vi "Sequence Status.vi"(5 "Exists Locally":bool, 7 "Local Error":bool, 10 "Local CRC":u32, 11 "Sequence Status JSON":T2) -> (3 "Sequence Status":T1=enum."Unloaded")   [LabVIEW 2023, in "VolatusSeqGUI.lvlib" / "Sequencing Control.lvclass"]
uses:
  Sequencing Control.lvclass
  VolatusSeq/Sequence Status JSON.ctl
  Sequence Status.ctl
  Sequencing Control.lvclass/Sequencing Control.ctl
  VolatusSeq/VolatusSeq.lvlib
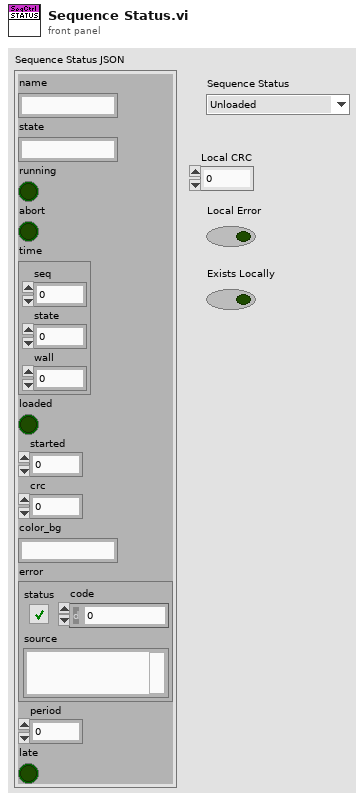
[diagram p1: front panel]
types:
  T1 = typedef "VolatusSeqGUI.lvlib/Sequencing Control.lvclass/Sequence Status.ctl" = enum16{"Unloaded Not Local", "Unloaded", "Load Error", "Loaded Good CRC", "Loaded Bad CRC", "Running Good CRC", "Running Bad CRC", "Local Error"}
  T2 = typedef "VolatusSeq.lvlib/Sequence Status JSON.ctl" = cluster{"name":string, "state":string, "running":bool, "abort":bool, "time":cluster{"seq":i64, "state":i64, "wall":i64}, "loaded":bool, "started":i64, "crc":u32, "color_bg":string, "error":errorcluster, "period":i64, "late":bool}
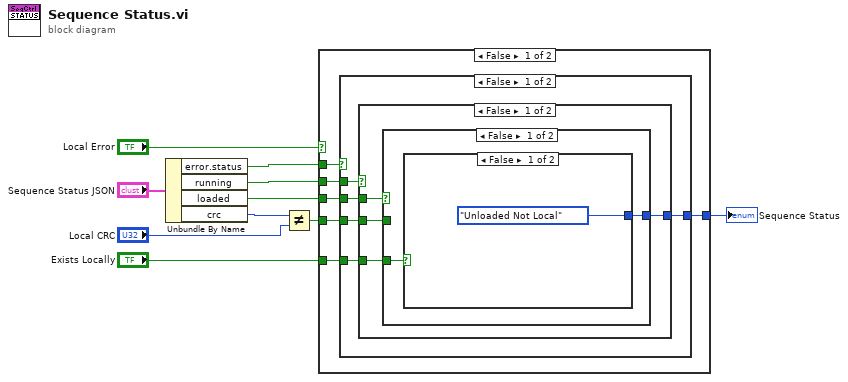
[diagram p0: block diagram]
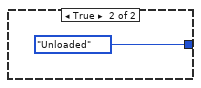
[diagram p2: hidden frame]
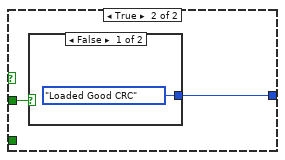
[diagram p3: hidden frame]
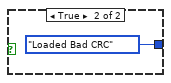
[diagram p4: hidden frame]
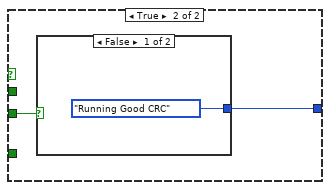
[diagram p5: hidden frame]
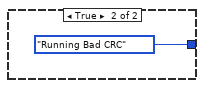
[diagram p6: hidden frame]
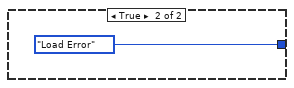
[diagram p7: hidden frame]
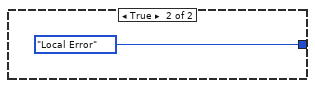
[diagram p8: hidden frame]
diagram:
  n1 = Unbundle By Name("Sequence Status JSON") -> ("error.status"=w3:bool, "running"=w6:bool, "loaded"=w7:bool, "crc"=w8:u32)
  n2 = Not Equal?(x=w8, y="Local CRC") -> (x != y?=w5:bool)
  n3 = case shown="False" "Local Error" {
    tunnel: w7 -> [w16 _]
    tunnel: w6 -> [w15 _]
    tunnel: w5 -> [w14 _]
    tunnel: [w13 Sequence_Status."Local Error" ("Sequence Status")] -> w4
    tunnel: w3 -> [w12 _]
    tunnel: "Exists Locally" -> [w11 _]
    frame False {
      n4 = case shown="False" w12 {
        tunnel: w16 -> [w21 _]
        tunnel: w15 -> [w20 _]
        tunnel: w14 -> [w19 _]
        tunnel: [w18 Sequence_Status."Load Error" ("Sequence Status")] -> w13
        tunnel: w11 -> [w17 _]
        frame False {
          n5 = case shown="False" w20 {
            tunnel: w21 -> [w25 _]
            tunnel: w19 -> [w24 w35]
            tunnel: [w23 w34] -> w18
            tunnel: w17 -> [w22 _]
            frame False {
              n6 = case shown="False" w25 {
                tunnel: w24 -> [_ w31]
                tunnel: [w27 w30] -> w23
                tunnel: w22 -> [w26 _]
                frame False {
                  n7 = case shown="False" w26 {
                    tunnel: [Sequence_Status."Unloaded Not Local" ("Sequence Status") Sequence_Status."Unloaded" ("Sequence Status")] -> w27
                    frame False {
                    }
                    frame True {
                    }
                  }
                }
                frame True {
                  n8 = case shown="False" w31 {
                    tunnel: [Sequence_Status."Loaded Good CRC" ("Sequence Status") Sequence_Status."Loaded Bad CRC" ("Sequence Status")] -> w30
                    frame False {
                    }
                    frame True {
                    }
                  }
                }
              }
            }
            frame True {
              n9 = case shown="False" w35 {
                tunnel: [Sequence_Status."Running Good CRC" ("Sequence Status") Sequence_Status."Running Bad CRC" ("Sequence Status")] -> w34
                frame False {
                }
                frame True {
                }
              }
            }
          }
        }
        frame True {
        }
      }
    }
    frame True {
    }
  }
  "Sequence Status" <- w4
